vi "Init.vi"(8 "error in (no error)":errorcluster, 11 "reference in":refnum<class "Switch_Keysight_34934A.lvclass">) -> (0 "error out":errorcluster, 3 "reference out":refnum<class "Switch_Keysight_34934A.lvclass">)   [LabVIEW 2022 SP3, in "Switch_Keysight_34934A.lvlib" / "Switch_Keysight_34934A.lvclass"]
uses:
  Switch_Keysight_34934A.lvclass
  Components/SwitchBase.lvlibp/SwitchBase.lvclass
  Components/ViPER.lvlibp/ViPER.lvclass
  C:/Projects/Medulla/ViPER/Examples/Flux_Capacitor_Tester/Components/ViPER.lvlibp/ViPER.lvclass
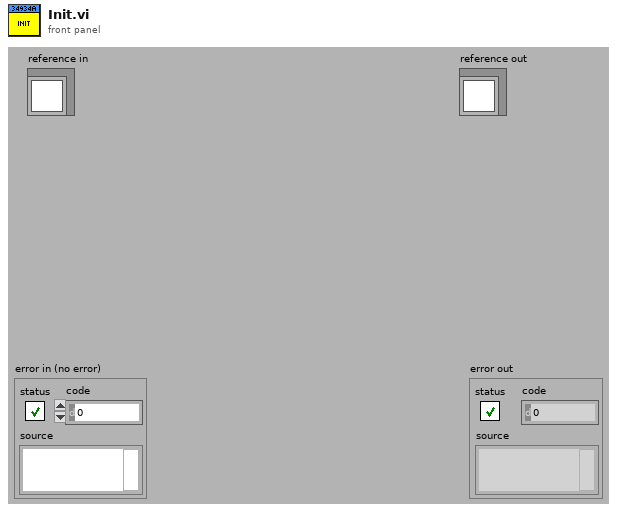
[diagram p1: front panel]
types:
  T1 = typedef "Switch_Keysight_34934A.lvlib/Switch_Keysight_34934A.lvclass/ObjectAttributes.ctl" = cluster{"Config":T2, "VISA ref":refnum<visa-resource-name>, "M1H":bool[][], "M2H":bool[][], "M1L":bool[][], "M2L":bool[][], "route":string, "State":bool[], "StateModBit":bool[], "UpdateEvent":refnum<user-event>}
  T2 = typedef "Switch_Keysight_34934A.lvlib/Switch_Keysight_34934A.lvclass/Config.ctl" = cluster{"VISA":refnum<visa-resource-name>, "Slot":i32, "SwitchMap":cluster{"Name":string, "Route":string[], "UnRoute":string[], "Description":string, "Group":string, "IsGroup":bool}[], "Sim":bool}
  T3 = cluster{"Name":string, "Route":string[], "UnRoute":string[], "Description":string, "Group":string, "IsGroup":bool}[]
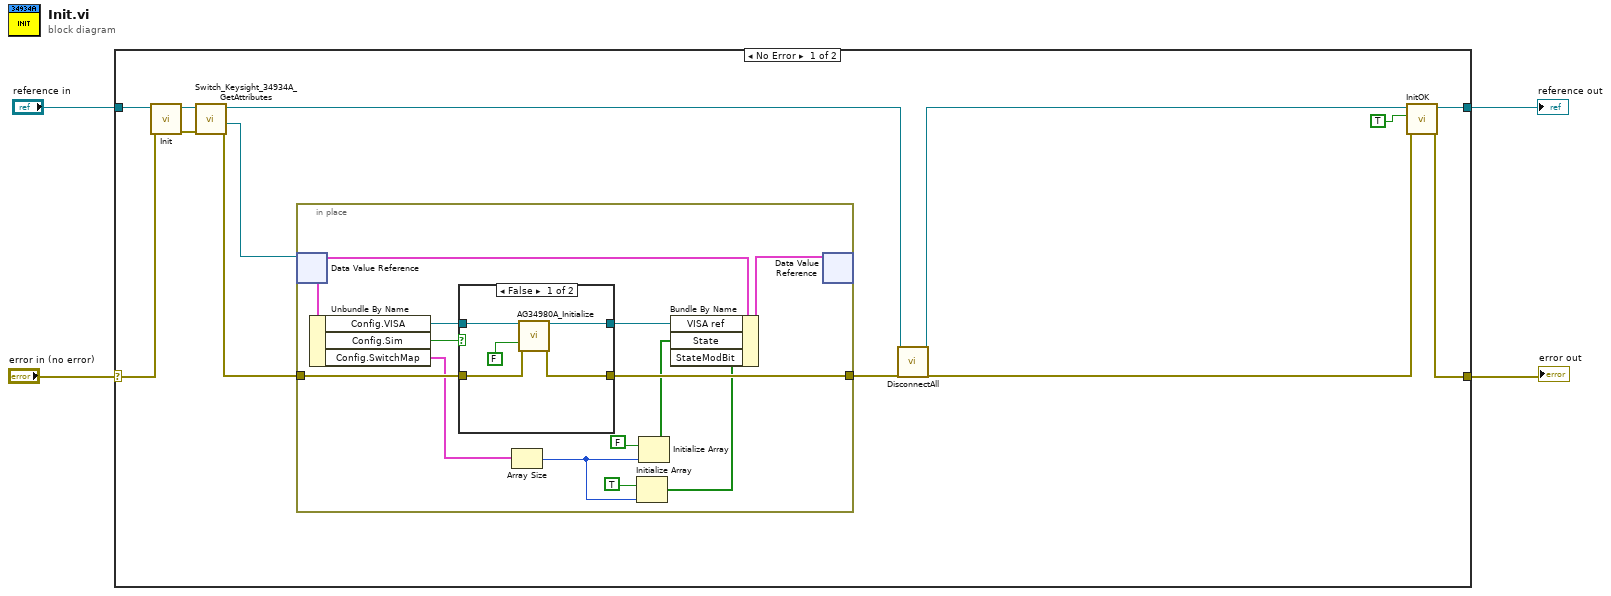
[diagram p0: block diagram]
diagram:
  n1 = case shown="No Error" "error in (no error)" {
    selector: "error in (no error)" -> [w16 w39]
    tunnel: [w9 w39] -> w3
    tunnel: [w11 w38] -> w1
    tunnel: "reference in" -> [w17 w38]
    frame No Error {
      n2 = call-parent "Init.vi"("error in (no error)"=w16, "reference in"=w17) -> ("error out"=w14:errorcluster, "reference out"=w15:refnum<class "Switch_Keysight_34934A.lvclass">)  [unwired: 8 in]
      n3 = call "Switch_Keysight_34934A_GetAttributes.vi"("error in (no error)"=w14, "reference in"=w15) -> ("error out"=w12:errorcluster, "DataRef"=w13:refnum<data-value>, "reference out"=w7:refnum<class "Switch_Keysight_34934A.lvclass">)  [unwired: 6 in, 1 out]
      n4 = in-place {
        in-place-border: w12 -> [w28]
        in-place-border: [w27] -> w8
        n5 = in-place-dvr #1(w13) -> (w30:T1)  [unwired: 1 out]
        n6 = Unbundle By Name(w30) -> ("Config.VISA"=w26:refnum<visa-resource-name>, "Config.Sim"=w24:bool, "Config.SwitchMap"=w23:T3)
        n7 = case shown="False" w24 {
          tunnel: w28 -> [w35 w37]
          tunnel: [w34 w37] -> w27
          tunnel: w26 -> [w33 w36]
          tunnel: [w32 w36] -> w25
          frame False {
            n8 = call "AG34980A_Initialize.vi"("VISA resource name"=w33, "Reset (True)"=FALSE, "error in (no error)"=w35) -> ("VISA session"=w32:refnum<visa-resource-name>, "error out"=w34:errorcluster)  [unwired: 11 in]
          }
          frame True {
          }
        }
        n9 = Array Size(array=w23) -> (size(s)=w19:i32)
        n10 = Initialize Array(TRUE, w19) -> (w18:bool[])
        n11 = Initialize Array(FALSE, w19) -> (w21:bool[])
        n12 = Bundle By Name(cluster=w30, "VISA ref"=w25, "State"=w21, "StateModBit"=w18) -> (w29:T1)
        n13 = in-place-dvr #1(w29) -> ()  [unwired: 2 out]
      }
      n14 = call-dynamic "DisconnectAll.vi"("reference in"=w7, "error in (no error)"=w8) -> ("reference in"=w6:refnum<class "Switch_Keysight_34934A.lvclass">, "error out"=w5:errorcluster)  [unwired: 16 in]
      n15 = call "InitOK.vi"("error in (no error)"=w5, "Init OK?"=TRUE, "reference in"=w6) -> ("error out"=w9:errorcluster, "reference out"=w11:refnum<class "Switch_Keysight_34934A.lvclass">)  [unwired: 7 in]
    }
    frame Error {
    }
  }
  "error out" <- w3
  "reference out" <- w1
